vi "Add Postprocessor.vi"(8 "error in (no error)":errorcluster, 9 "Reset":bool, 10 "Item Names":string[](array[string]), 11 "Monitor-Pulse in":refnum<class "Monitor-Pulse.lvclass">) -> (0 "error out":errorcluster, 3 "Monitor-Pulse out":refnum<class "Monitor-Pulse.lvclass">)   [LabVIEW 2016, in "Monitor-Pulse.lvclass"]
uses:
  Monitor-Pulse.lvclass
  Monitor-Pulse.lvclass/Monitor-Pulse.ctl
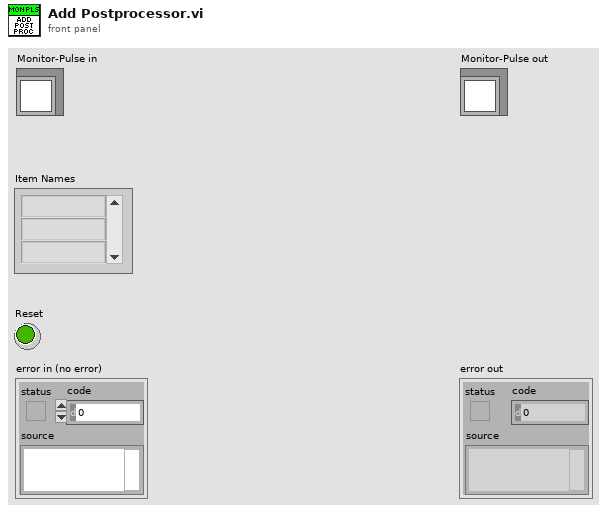
[diagram p1: front panel]
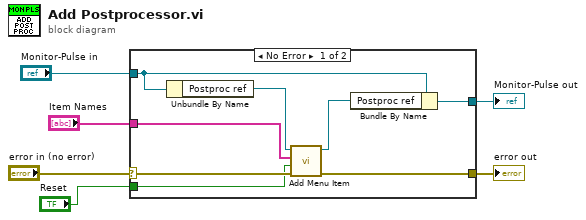
[diagram p0: block diagram]
diagram:
  n1 = case shown="No Error" "error in (no error)" {
    selector: "error in (no error)" -> [w9 w16]
    tunnel: [w11 w16] -> w5
    tunnel: [w10 w15] -> w3
    tunnel: "Monitor-Pulse in" -> [w13 w15]
    tunnel: "Item Names" -> [w8 _]
    tunnel: "Reset" -> [w7 _]
    frame No Error {
      n2 = Unbundle By Name(w13) -> ("Postproc ref"=w14:refnum<vi>)
      n3 = call "Add Menu Item.vi"("error in (no error)"=w9, "Reset"=w7, "Item Names"=w8, "Queed Listbox ref"=w14) -> ("error out"=w11:errorcluster, "Queed Listbox ref out"=w12:refnum<vi>)  [unwired: 5 in, 1 out]
      n4 = Bundle By Name(cluster=w13, "Postproc ref"=w12) -> (w10:refnum<class "Monitor-Pulse.lvclass">)
    }
    frame Error {
    }
  }
  "error out" <- w5
  "Monitor-Pulse out" <- w3
